vi "Enable Output.vi"(7 "Output Enabled (T: Enable)":bool=TRUE, 8 "error in (no error)":errorcluster, 11 "VISA resource name":refnum<visa-resource-name>) -> (0 "error out":errorcluster, 3 "VISA resource name out":refnum<visa-resource-name>)   [LabVIEW 2012, in "Fluke 5080.lvlib"]
doc: "Enables or disables the calibration output."
uses:
  <instrlib>/Fluke 5080/Fluke 5080.lvlib
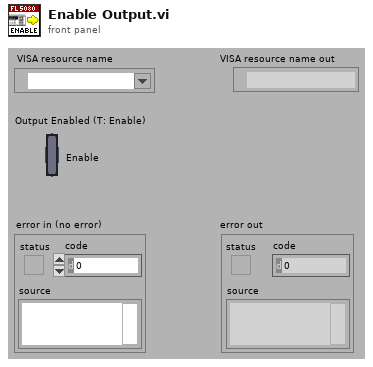
[diagram p1: front panel]
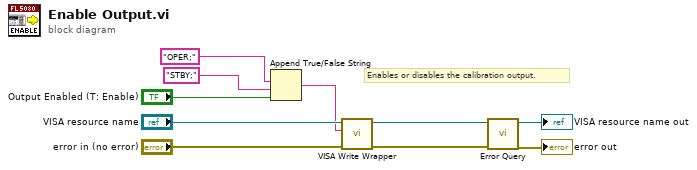
[diagram p0: block diagram]
diagram:
  # "Enables or disables the calibration output."
  n1 = Append True/False String(1:"Output Enabled (T: Enable)", 2:"STBY;", 3:"OPER;") -> (0:w5:string)  [unwired: 1 out]
  n2 = call <instrlib>:"VISA Write Wrapper.vi"("error in (no error)"="error in (no error)", "Write Buffer"=w5, "VISA resource name"="VISA resource name") -> ("error out"=w1:errorcluster, "VISA resource name out"=w2:refnum<visa-resource-name>)  [unwired: 7 out]
  n3 = call <instrlib>:"Error Query.vi"("error in (no error)"=w1, "VISA resource name"=w2) -> ("error out"=→"error out":errorcluster, "VISA resource name out"=→"VISA resource name out":refnum<visa-resource-name>)  [unwired: 8 out]
